vi "Data JSON.vi"(8 "error in (no error)":errorcluster, 11 "Request in":refnum<class "Request.lvclass">) -> (0 "error out":errorcluster, 2 "Data JSON":string, 3 "Request out":refnum<class "Request.lvclass">)   [LabVIEW 2020, in "obs-websocket.lvlib" / "Request.lvclass"]
uses:
  Request.lvclass
  Request.lvclass/Request.ctl
  81c80b76-1bed-4b65-a226-f010383d1a8a.vi
  f0dcadc8-9197-4ea2-8fdd-3128689d0f4b.vi
  <vilib>/JDP Science/JSONtext/Variant to JSON Text.vi
  <vilib>/JDP Science/JSONtext/LVClass Serializer/JSONtext LVClass Serializer.lvclass
  <vilib>/JDP Science/JSONtext/JSONtext.lvlib
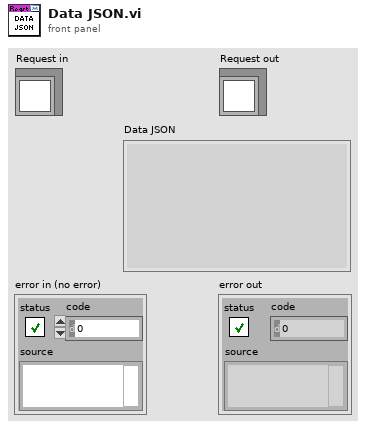
[diagram p1: front panel]
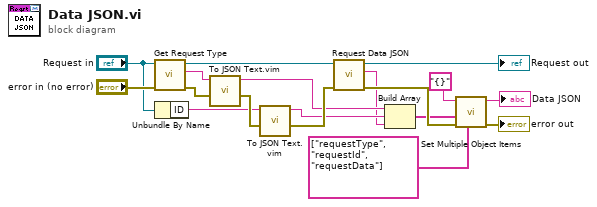
[diagram p0: block diagram]
diagram:
  n1 = call-dynamic "Get Request Type.vi"("error in (no error)"="error in (no error)", "Request in"="Request in") -> ("error out"=w12:errorcluster, "Request Type"=w13:string, "Request out"=w16:refnum<class "Request.lvclass">)  [unwired: 7 in]
  n2 = Unbundle By Name("Request in") -> ("ID"=w9:string)
  n3 = call "To JSON Text.vim"("error in (no error)"=w12, "Anything"=w13) -> ("error out"=w10:errorcluster, "<JSON>"=w7:string)  [unwired: 8 in]
  n4 = call "To JSON Text.vim"("error in (no error)"=w10, "Anything"=w9) -> ("error out"=w8:errorcluster, "<JSON>"=w6:string)  [unwired: 8 in]
  n5 = call-dynamic "Request Data JSON.vi"("error in (no error)"=w8, "Request in"=w16) -> ("error out"=w18:errorcluster, "Request Data JSON"=w1:string, "Request out"=→"Request out":refnum<class "Request.lvclass">)  [unwired: 7 in]
  n6 = Build Array(w7, w6, w1) -> (w5:string[])
  n7 = call <vilib>:"Set Multiple Object Items.vi"("Item Names"=string[] ["requestType", "requestId", "requestData"], "error in (no error)"=w18, "JSON Items"=w5, "JSON"="{}") -> ("error out"=→"error out":errorcluster, "<JSON>"=→"Data JSON":string)  [unwired: 5 in]
